vi "Is Initialized.vi"(8 "error in":errorcluster, 11 "gRPC XNET Read Raw CAN Frame Strategy in":refnum<class "gRPC XNET Read Raw CAN Frame Strategy.lvclass">) -> (0 "error out":errorcluster, 2 "Is Initialized?":bool, 3 "gRPC XNET Read Raw CAN Frame Strategy out":refnum<class "gRPC XNET Read Raw CAN Frame Strategy.lvclass">)   [LabVIEW 2024, in "gRPC XNET Read Raw CAN Frame Strategy.lvclass"]
uses:
  gRPC XNET Read Raw CAN Frame Strategy.lvclass
  gRPC XNET Read Raw CAN Frame Strategy.lvclass/gRPC XNET Read Raw CAN Frame Strategy.ctl
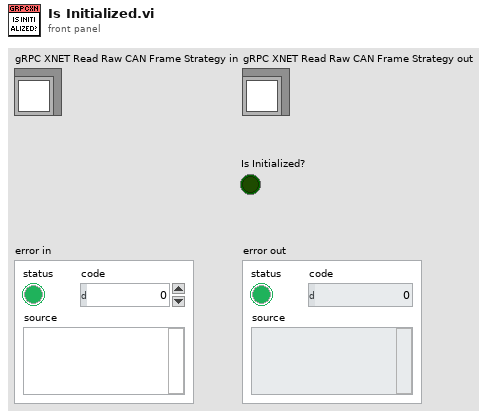
[diagram p1: front panel]
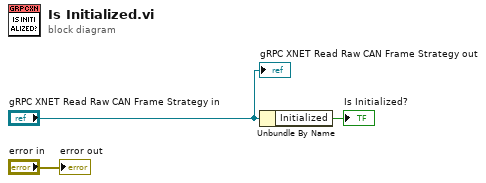
[diagram p0: block diagram]
diagram:
  n1 = Unbundle By Name("gRPC XNET Read Raw CAN Frame Strategy in") -> ("Initialized"=→"Is Initialized?":bool)
  "gRPC XNET Read Raw CAN Frame Strategy out" <- "gRPC XNET Read Raw CAN Frame Strategy in"
  "error out" <- "error in"
